vi "UDP Multicast - Receiver.vi"() -> ()   [LabVIEW 2014]
doc: "创建一个只读UDP多点传送会话并接收指定端口的数据。"
uses:
  <vilib>/Utility/importsl/GetValueByPointer/datatype.ctl
  <vilib>/Utility/tcp.llb/UDP Multicast Read-Only Open.vi
  <vilib>/Utility/importsl/GetValueByPointer/GetValueByPointer.xnode
  <vilib>/regexp/Match Regular Expression.xnode
  FromWSY/dll/AriaDll.dll
panel:
  out "数值 4":dbl
  out "数值 3":dbl
  out "x < y?":bool
  out "返回类型 3":i32
  out "poseY":i32
  out "poseX":i32
  out "元素 2":dbl
  out "元素":dbl
  out "数值 2":dbl
  in  "数组 2":dbl[][](array[numeric])
  out "Path 2":string[](array[string])
  out "Area 3":string[](array[string])
  out "Dis 2":dbl
  out "Path坐标数组":dbl[][](array[numeric])
  out "standard error":string caption="标准错误"
  out "error out":errorcluster caption="错误输出"
  out "数组":string[][](array[string])
  out "字符串 2":string
  out "Voltage":dbl
  out "RotVel":dbl
  out "LatVel":dbl
  out "Vel":dbl
  out "Th":dbl
  out "Y":dbl
  out "X":dbl
  out "返回类型 2":i32
  out "Status":string
  out "Mode":string
  out "返回类型":i32
  in  "停止":bool
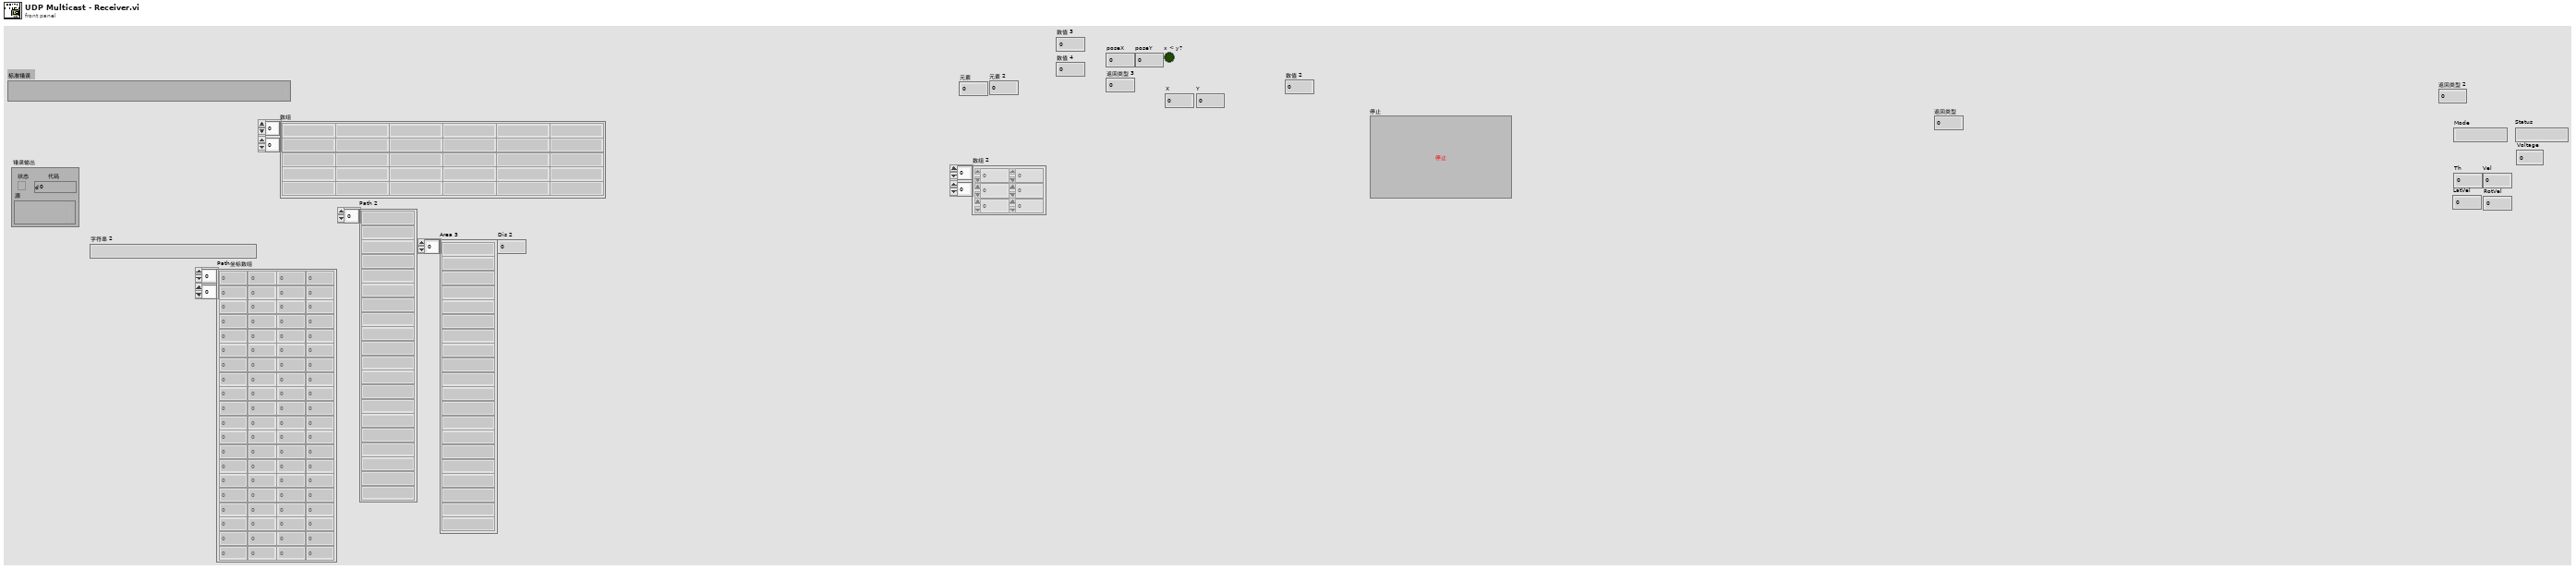
[diagram p1: front panel]
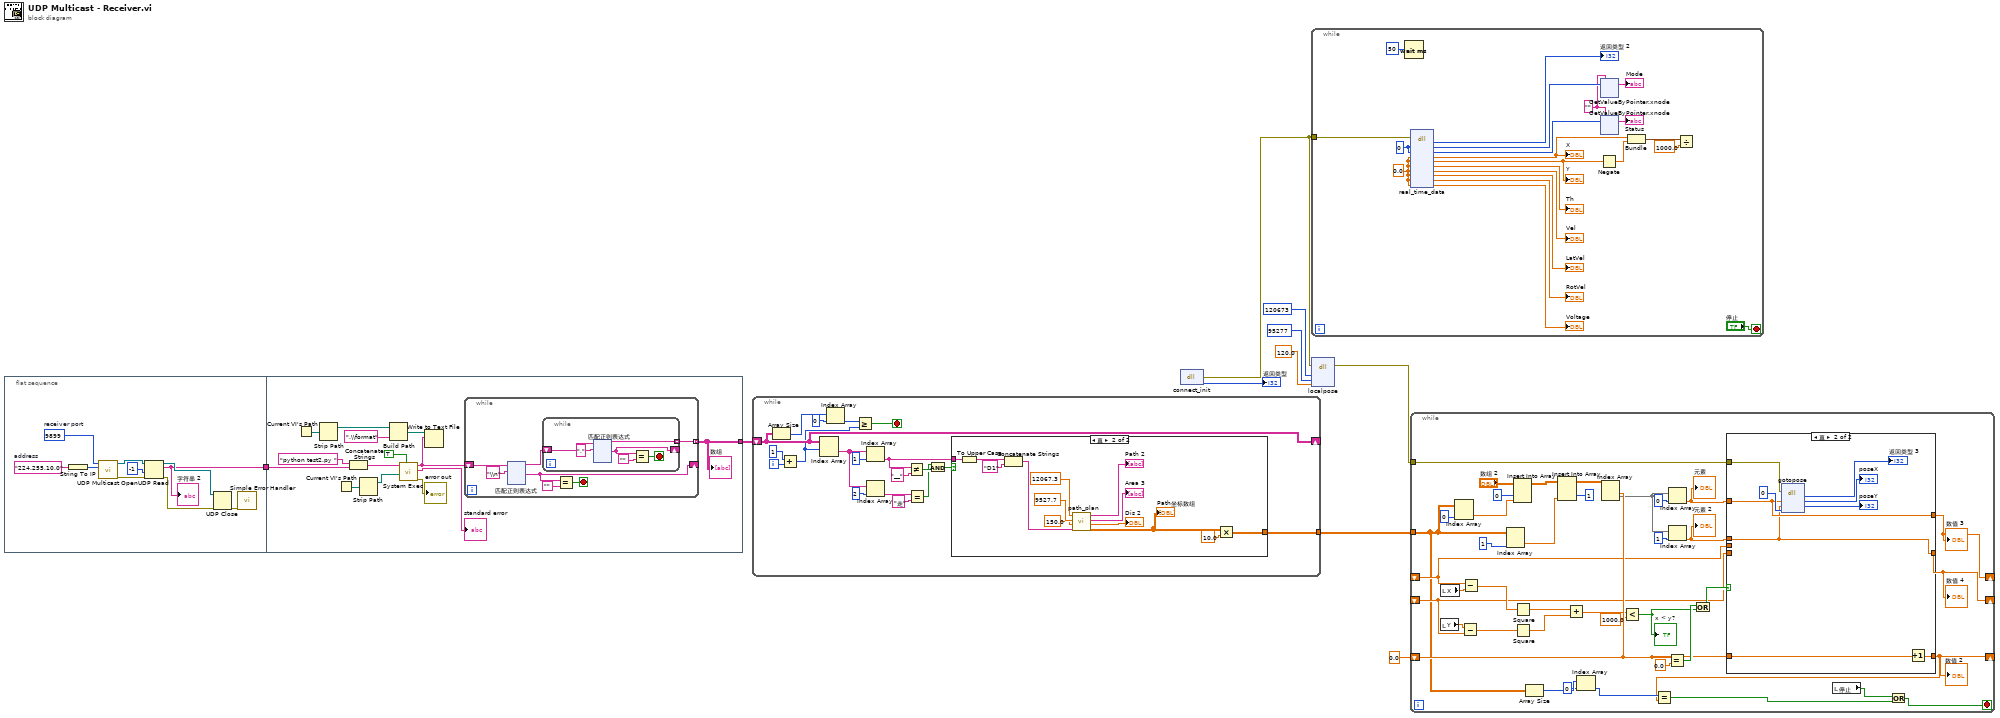
[diagram p0: block diagram]
diagram:
  n1 = flat-sequence {
    tunnel: [w11] -> w4
    tunnel: w4 -> [w27]
    tunnel: [w21] -> w3
    frame #0 {
      w13 = u16 9899  # receiver port
      w12 = "224.255.10.0"  # address
      n2 = String To IP(1:w12) -> (0:w14:u32)
      n3 = call-poly <vilib>:"UDP Multicast Open.vi"("multicast addr"=w14, "port"=w13) -> ("error out"=w19:errorcluster, "connection ID"=w16:refnum<k16>)  [unwired: 7 in, 1 out]
      n4 = UDP Read(connection ID=w16, timeout ms (25000)=-1, 8:w19) -> (data out=w11:string, error out=w20:errorcluster, 3:w18:refnum<k16>)  [unwired: 3 out]
      "字符串 2" <- w11
      n5 = UDP Close(connection ID=w18, 8:w20) -> (error out=w17:errorcluster)  [unwired: 1 out]
      n6 = call <vilib>:"Simple Error Handler.vi"("error in (no error)"=w17) -> ()  [unwired: 1 in, 8 out]
    }
    frame #1 {
      n7 = Current VI's Path() -> (path=w26:path)
      n8 = Strip Path(path=w26) -> (stripped path=w25:path)  [unwired: 1 out]
      n9 = Current VI's Path() -> (path=w30:path)
      n10 = Concatenate Strings("python test2.py " ("command line"), w27) -> (w28:string)
      n11 = Strip Path(path=w30) -> (stripped path=w31:path)  [unwired: 1 out]
      n12 = Build Path(base path=w25, name or relative path=".\\format" ("名称或相对路径")) -> (appended path=w23:path)
      n13 = call <vilib>:"System Exec.vi"("wait until completion? (T)"=TRUE, "working directory"=w31, "command line"=w28) -> ("error out"=→"error out":errorcluster, "standard error"=→"standard error":string, "standard output"=w22:string)  [unwired: 5 in, 1 out]
      n14 = Write to Text File(file (use dialog)=w23, text=w22) -> ()  [unwired: 2 in, 3 out]
      n15 = while {
        tunnel: [w35] -> w21 mode=indexing
        shift-right: [w39] -> _
        shift-left: w22 -> [w40]
        stop <- w37 stop-if-true
        n16 = xnode "匹配正则表达式"("输入字符串"=w40, "正则表达式"="\\n") -> ("匹配之前"=w36:string, "匹配之后"=w39:string)  [unwired: 4 in, 3 out]
        n17 = while {
          shift-right: [w43] -> _
          shift-left: w36 -> [w47]
          tunnel: [w45] -> w35 mode=indexing
          stop <- w42 stop-if-true
          n18 = xnode "匹配正则表达式"("输入字符串"=w47, "正则表达式"=",") -> ("匹配之前"=w45:string, "匹配之后"=w43:string)  [unwired: 4 in, 3 out]
          n19 = Equal?(x=w43, y="") -> (x = y?=w42:bool)
        }
        n20 = Equal?(x=w39, y="") -> (x = y?=w37:bool)
      }
      "数组" <- w21
    }
  }
  n21 = while {
    shift-right: [w290] -> _
    shift-left: w3 -> [w290]
    tunnel: [w276] -> w2
    i -> [w292]
    stop <- w289 stop-if-true
    n22 = Array Size(array=w290) -> (size(s)=w294:i32[])
    n23 = Add(x=1, y=w292) -> (x+y=w287:i32)
    n24 = Index Array(array=w290, index (row)=w287) -> (element=w282:string[])  [unwired: 1 in]
    n25 = Index Array(array=w294, index=0 ("索引")) -> (element=w288:i32)
    n26 = Greater Or Equal?(x=w288, y=w287) -> (x >= y?=w289:bool)
    n27 = Index Array(array=w282, index=1 ("索引")) -> (element=w277:string)
    n28 = Index Array(array=w282, index=2 ("索引")) -> (element=w285:string)
    n29 = Not Equal?(x=w277, y="__") -> (x != y?=w280:bool)
    n30 = Equal?(x=w285, y="走") -> (x = y?=w279:bool)
    n31 = And(x=w279, y=w280) -> (x .and. y?=w278:bool)
    n32 = case shown="真" w278 {
      tunnel: w277 -> [_ w307]
      tunnel: [_ w296] -> w276
      frame False {
      }
      frame True {
        n33 = To Upper Case(1:w307) -> (0:w306:string)
        n34 = Concatenate Strings(w306, "D1" ("字符串")) -> (w304:string)
        n35 = call "path_plan.vi"("Node2"=w304, "z"=150.0, "y"=9527.7, "x"=12067.3) -> ("Path坐标数组"=w297:dbl[][], "Dis 2"=→"Dis 2":dbl, "Area 3"=→"Area 3":string[], "Path 2"=→"Path 2":string[])
        "Path坐标数组" <- w297
        n36 = Multiply(x=w297, y=10.0) -> (x*y=w296:dbl[][])
      }
    }
  }
  n37 = dll-call lib="E:/labview/1511/zsControlSystem2.0/FromOtherProject/FromWSY/dll/AriaDll.dll" fn="connect_init"() -> (error out=w6:errorcluster, "返回类型"=→"返回类型":i32)  [unwired: 3 in, 1 out]
  n38 = while {
    tunnel: w6 -> [w308]
    stop <- "停止" stop-if-true
    w320 = 0.0
    w322 = ""
    w324 = u64 0 ("Mode")
    n39 = Wait (ms)(milliseconds to wait=u32 50 ("毫秒计时值")) -> ()  [unwired: 1 out]
    n40 = dll-call lib="E:/labview/1511/zsControlSystem2.0/FromOtherProject/FromWSY/dll/AriaDll.dll" fn="real_time_data"(error in=w308, "Mode"=w324, "Status"=w324, "X"=w320, "Y"=w320, "Th"=w320, "Vel"=w320, "LatVel"=w320, "RotVel"=w320, "Voltage"=w320) -> ("返回类型"=→"返回类型 2":i32, "Mode"=w327:u64, "Status"=w323:u64, "X"=w313:dbl, "Y"=w312:dbl, "Th"=→"Th":dbl, "Vel"=→"Vel":dbl, "LatVel"=→"LatVel":dbl, "RotVel"=→"RotVel":dbl, "Voltage"=→"Voltage":dbl)  [unwired: 2 in, 2 out]
    "X" <- w313
    "Y" <- w312
    n41 = Negate(x=w312) -> (-x=w310:dbl)
    n42 = xnode "GetValueByPointer.xnode"("Pointer"=w327, "InputType"=w322) -> ("Output"=→"Mode":string)  [unwired: 2 in, 1 out]
    n43 = xnode "GetValueByPointer.xnode"("Pointer"=w323, "InputType"=w322) -> ("Output"=→"Status":string)  [unwired: 2 in, 1 out]
    n44 = Bundle("X"=w313, w310) -> (w311:cluster{"X":dbl, dbl})  [unwired: 1 in]
    n45 = Divide(x=w311, y=1000.0) -> ()  [unwired: 1 out]
  }
  n46 = dll-call lib="E:/labview/1511/zsControlSystem2.0/FromOtherProject/FromWSY/dll/AriaDll.dll" fn="localpose"(error in=w6, "LocalposeX"=120673, "LocalposeY"=95277, "LocalposeTh"=120.0) -> (error out=w5:errorcluster)  [unwired: 6 in, 1 out]
  n47 = while {
    tunnel: w5 -> [w384]
    tunnel: w2 -> [w360]
    shift-right: [w356] -> _
    shift-left: 0.0 ("数值") -> [w378]
    shift-right: [w364] -> _
    shift-left: _ -> [w361]
    shift-right: [w363] -> _
    shift-left: _ -> [w362]
    stop <- w353 stop-if-true
    n48 = local read "X"() -> (w375:dbl)
    n49 = local read "Y"() -> (w372:dbl)
    n50 = Index Array(array=w360, index (col)=0 ("禁用的索引 (列)")) -> (element=w388:dbl[])  [unwired: 1 in]
    n51 = Subtract(x=w372, y=w362) -> (x-y=w370:dbl)
    n52 = Subtract(x=w361, y=w375) -> (x-y=w373:dbl)
    n53 = Index Array(array=w360, index (col)=1 ("禁用的索引 (列)")) -> (element=w386:dbl[])  [unwired: 1 in]
    n54 = Insert Into Array(array="数组 2", index (col)=0 ("禁用的索引 (列)"), new element=w388) -> (w387:dbl[][])  [unwired: 1 in]
    n55 = Square(x=w373) -> (x^2=w369:dbl)
    n56 = Square(x=w370) -> (x^2=w368:dbl)
    n57 = Array Size(array=w360) -> (size(s)=w359:i32[])
    n58 = Insert Into Array(array=w387, index (col)=1 ("禁用的索引 (列)"), new element=w386) -> (w376:dbl[][])  [unwired: 1 in]
    n59 = Add(x=w369, y=w368) -> (x+y=w367:dbl)
    n60 = Index Array(array=w359, index=0 ("索引")) -> (element=w357:i32)
    n61 = Index Array(array=w376, index (row)=w378) -> (element=w377:dbl[])  [unwired: 1 in]
    n62 = Less?(x=w367, y=1000.0) -> (x < y?=w365:bool)
    "x < y?" <- w365
    n63 = Equal?(x=w378, y=0.0) -> (x = y?=w380:bool)
    n64 = Index Array(array=w377, index=0 ("索引")) -> (element=w374:dbl)
    "元素" <- w374
    n65 = Index Array(array=w377, index=1 ("索引")) -> (element=w371:dbl)
    "元素 2" <- w371
    n66 = Or(x=w380, y=w365) -> (x .or. y?=w379:bool)
    n67 = case shown="真" w379 {
      tunnel: w384 -> [_ w403]
      tunnel: w378 -> [w395 w399]
      tunnel: [w395 w396] -> w356
      tunnel: w374 -> [_ w398]
      tunnel: w371 -> [_ w397]
      tunnel: [w393 w398] -> w364
      tunnel: [w394 w397] -> w363
      tunnel: w362 -> [w394 _]
      tunnel: w361 -> [w393 _]
      frame False {
      }
      frame True {
        n68 = dll-call lib="E:/labview/1511/zsControlSystem2.0/FromOtherProject/FromWSY/dll/AriaDll.dll" fn="gotopose"(error in=w403, "poseX"=w398, "poseY"=w397, "poseTh"=0) -> ("返回类型"=→"返回类型 3":i32, "poseX"=→"poseX":i32, "poseY"=→"poseY":i32)  [unwired: 3 in, 2 out]
        n69 = Increment(x=w399) -> (x+1=w396:dbl)
      }
    }
    "数值 2" <- w356
    "数值 3" <- w364
    "数值 4" <- w363
    n70 = Equal?(x=w357, y=w356) -> (x = y?=w354:bool)
    n71 = local read "停止"() -> (w355:bool)
    n72 = Or(x=w355, y=w354) -> (x .or. y?=w353:bool)
  }
